vi "TestHB_Emb_1.vi"() -> ()   [LabVIEW 2012]
doc: "SciScan 1.2 160622"
uses:
  SubVIs/Heartbeat state manager Input VI names.ctl
  Custom Controls and Typedefs/HFG Commands.ctl
  Custom Controls/Heartbeat_States.ctl
  Custom Controls and Typedefs/HB Actionable Event.ctl
  Custom Controls and Typedefs/Heartbeat Event Source.ctl
  Custom Controls and Typedefs/Heartbeat information cluster.ctl
  SubVIs/Master Slave messaging Flags.ctl
  Custom Controls and Typedefs/HB_Error Conditions Cluster.ctl
panel:
  out "Commands Sent":i32
  out "No of slave confirmation":i32
  out "Error conditions Cluster":T1
  out "Master-Slave messaging Flags":T2={"Instruction available"=TRUE, "Slave action completed"=TRUE, "Slave Ready?"=FALSE}
  out "Heartbeat information cluster":T3
  in  "stop 3":bool
  in  "stop 2":bool
  out "Commands Issued":i32
  in  "Completion simulator":bool
  in  "Array":string[](array[string])=["Hi", "This", "Is", "A", "Test", "fg", "fgg", "ghg", "gh", "gh", "gh", "h", "hg", "f", "gn", "dghs", "dgh", "dghd", "dh", "d", "dghz", "afd", "gh", "afdg", "adfg", "dafg", "dfgh", "adfg", "dfg", "fdg", "dafg", "a", "hz", "fg", "dafg", "fdg", "adfg", "ag", "hadfg", "dfg", "adfg", "afg", "gjsgh", "dfhg", "dfg", "dfg", "jadfgh", "fhad", "hdgfh", "adfg", "hsdhgf", "adfg", "hdgfh", "fgg", "hdafh", "fdghfd", "hgsdha", "adfga", "ghadfh", "fdh", "fhjda", "fgasd", "hdha", "ahfdjhs", "dha", "hjg", "jgfsj", "adgh", "sdgh", "dsgjs", "adfh", "sdgha", "fdha", "dfhhs", "hgshjs", "gjhs", "gdh", "sgfh", "sgh", "gjhs", "hfdj", "dsfhj", "dfh", "jdhj", "fhjd", "ghfg", "fhjd", "dfjdf", "hjdf", "gjdfgj", "fhjd", "jkkg", "kfdh", "dfhjsd", "fhj", "fhj", "sfgj", "sfgjsf", "fgjgfj", "sfgjsf", "jfghjsgf", "fghjsf", "fsghj"]
  in  "Cancel simulator":bool
  out "Error Out":errorcluster
  in  "Error In":errorcluster
  in  "Command Issue simulator":bool
  in  "stop":bool
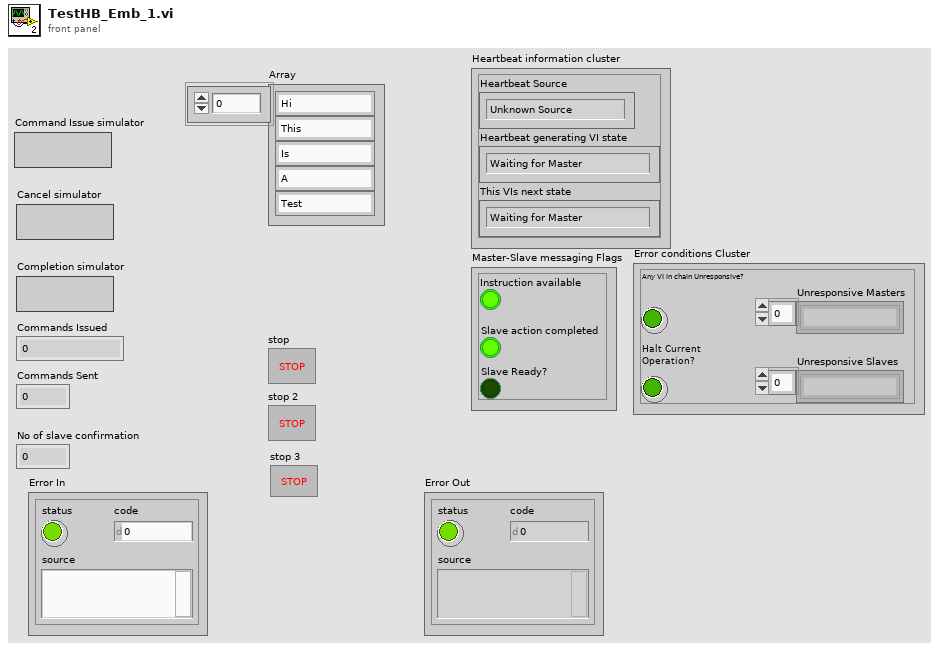
[diagram p1: front panel]
types:
  T1 = typedef "HB_Error Conditions Cluster.ctl" = cluster{"Any VI in chain Unresponsive?":bool, "Halt Current Operation?":bool, "Unresponsive Masters":string[], "Unresponsive Slaves":string[]}
  T2 = typedef "Master Slave messaging Flags.ctl" = cluster{"Instruction available":bool, "Slave action completed":bool, "Slave Ready?":bool}
  T3 = typedef "Heartbeat information cluster.ctl" = cluster{"Heartbeat Source":T4, "Heartbeat generating VI state":T5, "This VIs next state":T5}
  T4 = typedef "Heartbeat Event Source.ctl" = enum16{"Unknown Source", "Timeout", "This VI", "Master", "Slave"}
  T5 = typedef "Heartbeat_States.ctl" = enum16{"Waiting for Master", "Instruction Issued", "Waiting for Slave Completion", "Completed", "Cancelled", "Failed", "Broken Link"}
  T6 = enum8{"Enabled", "Disabled", "Disabled and Grayed Out"}
  T7 = typedef "HB Actionable Event.ctl" = enum16{"Master instruction event", "Slave ready event", "Slave unavailable event", "Cancelled or Failed event", "Slave action complete event", "QUIT", "Broken Link", "Recovered from Broken Link"}
  T8 = typedef "Heartbeat state manager Input VI names.ctl" = cluster{"Current VI name":string, "Master VI Names":string[], "Slave VI Names":string[]}
  T9 = typedef "HFG Commands.ctl" = enum16{"Set", "Get", "Initialize"}
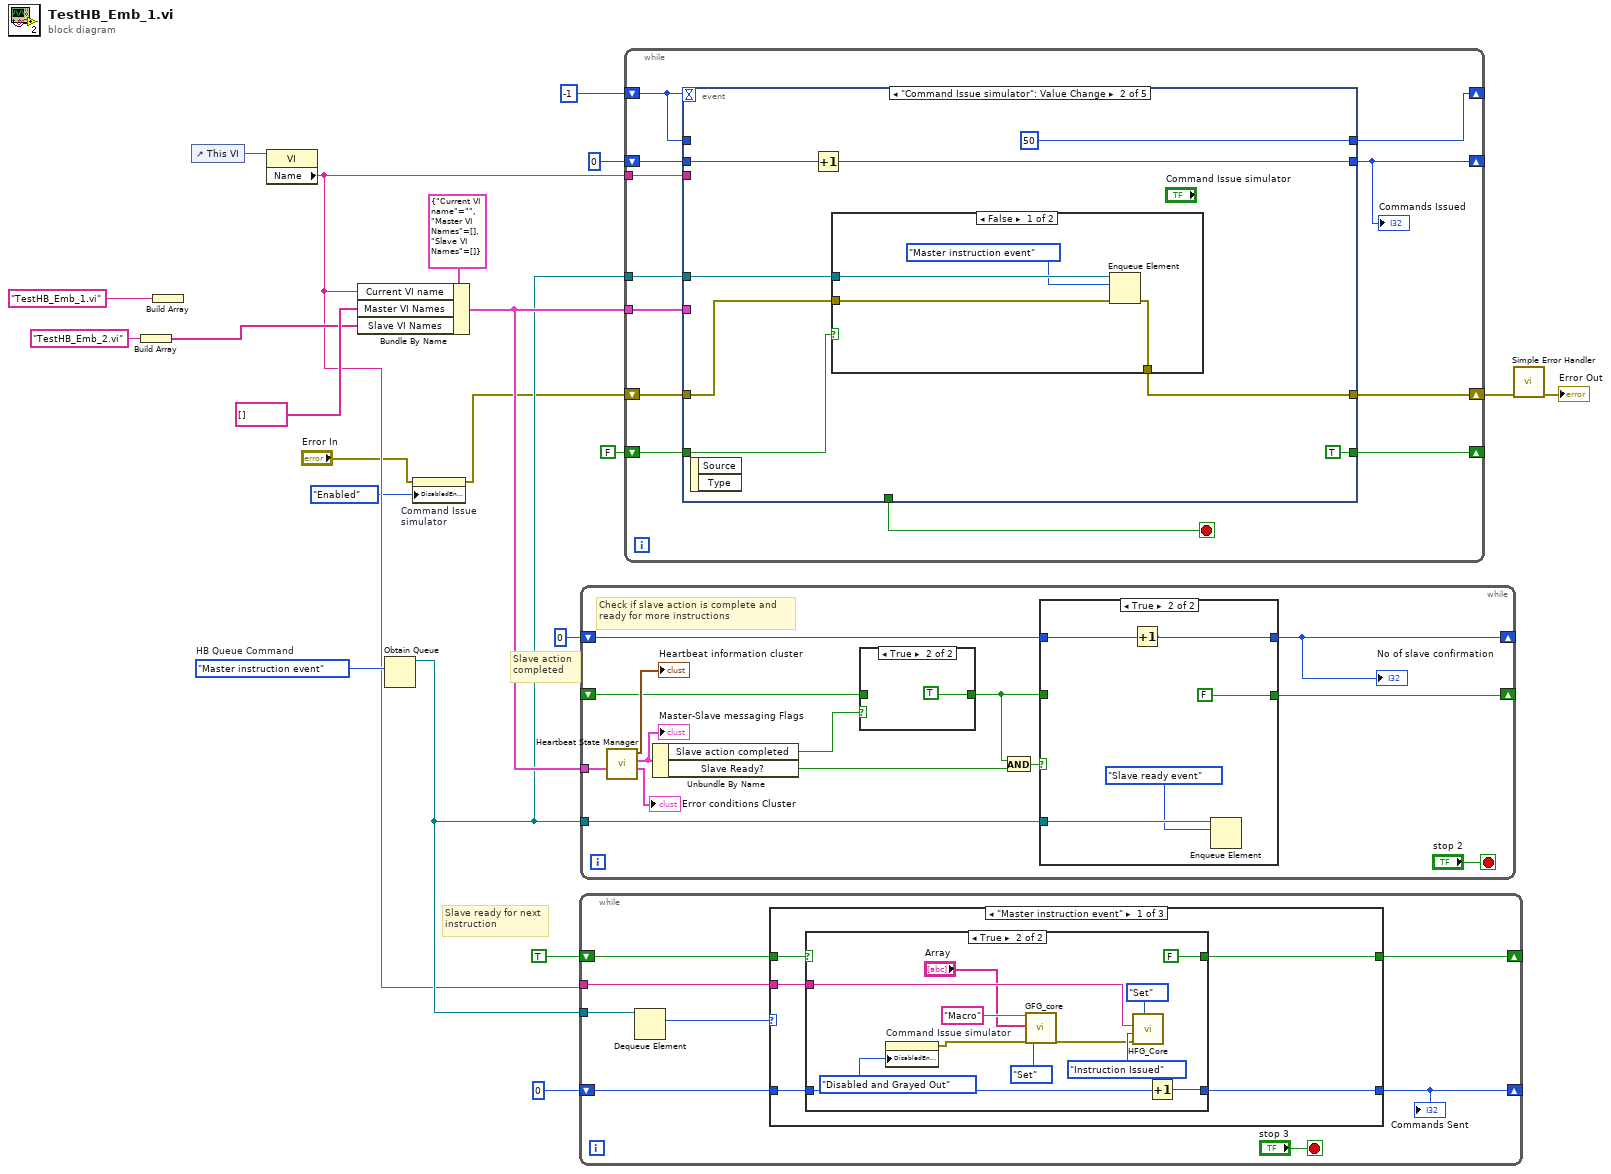
[diagram p0: block diagram]
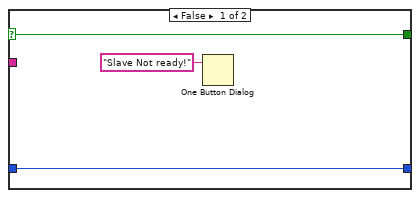
[diagram p2: hidden frame]
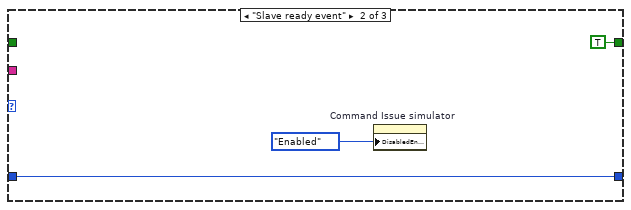
[diagram p3: hidden frame]
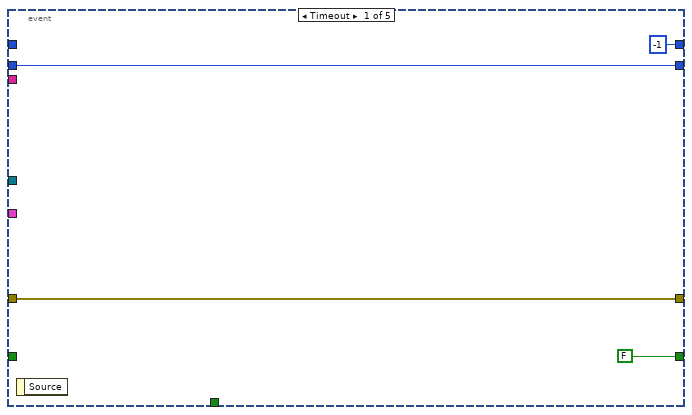
[diagram p7: hidden frame]
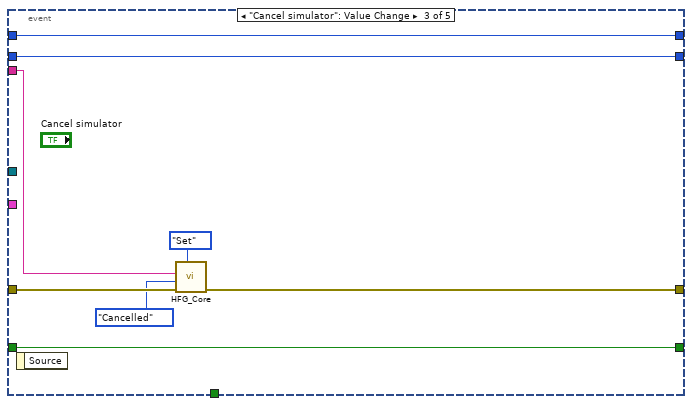
[diagram p9: hidden frame]
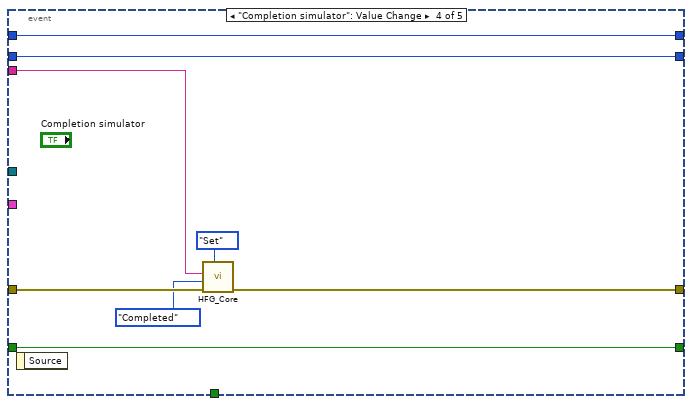
[diagram p10: hidden frame]
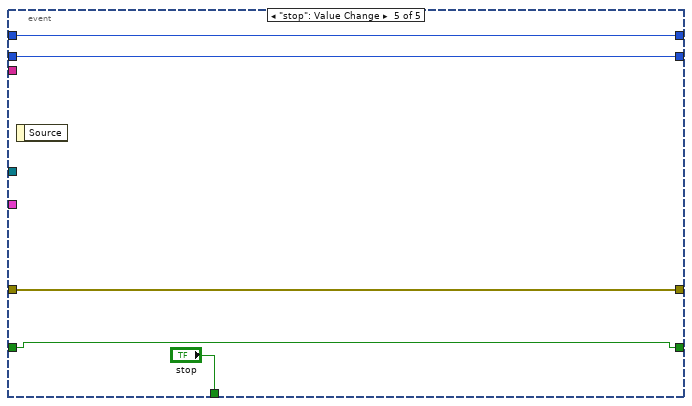
[diagram p11: hidden frame]
diagram:
  w12 = HB_Actionable_Event."Master instruction event"  # HB Queue Command
  # "Slave action \ncompleted"
  # "Slave ready for next\ninstruction"
  n1 = Build Array("TestHB_Emb_2.vi") -> (w17:string[])
  n2 = Build Array("TestHB_Emb_1.vi") -> ()  [unwired: 1 out]
  n3 = control-ref of="This VI"() -> (w16:refnum<vi>)
  n4 = property class="VI"(reference=w16) -> ("Name"=w10:string)  [unwired: 1 in, 2 out]
  n5 = Bundle By Name(cluster=T8 {"Current VI name"="", "Master VI Names"=[], "Slave VI Names"=[]} ("Heartbeat state manager Input VI names 2"), "Current VI name"=w10, "Master VI Names"=string[] [], "Slave VI Names"=w17) -> (w13:T8)
  n6 = Obtain Queue(element data type=w12) -> (queue out=w11:refnum<queue>)  [unwired: 4 in, 2 out]
  n7 = property on="Command Issue simulator" class="Bool"(error in="Error In", "DisabledEnum"=T6."Enabled" ("Disabled")) -> (error out=w7:errorcluster)  [unwired: 1 in, 1 out]
  n8 = while {
    tunnel: w11 -> [w29]
    tunnel: w10 -> [w26]
    shift-right: [w25] -> _
    shift-left: TRUE -> [w24]
    shift-right: [w22] -> _
    shift-left: 0 -> [w23]
    stop <- "stop 3" stop-if-true
    n9 = Dequeue Element(queue=w29) -> (element=w28:T7)  [unwired: 2 in, 3 out]
    n10 = case shown="\"Master instruction event\"" w28 {
      tunnel: w26 -> [w34 _ _]
      tunnel: [w32 TRUE w54] -> w25
      tunnel: w24 -> [w33 _ w54]
      tunnel: w23 -> [w31 w50 w53]
      tunnel: [w30 w50 w53] -> w22
      frame "Master instruction event" {
        n11 = case shown="True" w33 {
          selector: w33 -> [w36 _]
          tunnel: w34 -> [_ w49]
          tunnel: [w36 FALSE] -> w32
          tunnel: w31 -> [w35 w39]
          tunnel: [w35 w38] -> w30
          frame False {
            n12 = One Button Dialog(message="Slave Not ready!") -> ()  [unwired: 1 in, 1 out]
          }
          frame True {
            n13 = property on="Command Issue simulator" class="Bool"("DisabledEnum"=T6."Disabled and Grayed Out" ("Disabled")) -> (error out=w40:errorcluster)  [unwired: 2 in, 1 out]
            n14 = call "GFG_core.vi"("Variable Name in"="Macro", "Variant in"="Array", "error in (no error)"=w40, "Action"=enum16{"Init", "Set", "Get", "Clear"}."Set") -> ("error out"=w46:errorcluster)  [unwired: 9 in, 6 out]
            n15 = call "HFG_Core.vi"("HFG Commands"=HFG_Commands."Set", "Error In"=w46, "Heartbeat state IN"=Heartbeat_States."Instruction Issued", "VI Name (Calling VIs name by default)"=w49) -> ()  [unwired: 4 in, 4 out]
            n16 = Increment(x=w39) -> (x+1=w38:i32)
          }
        }
      }
      frame "Slave ready event" {
        n17 = property on="Command Issue simulator" class="Bool"("DisabledEnum"=T6."Enabled" ("Disabled")) -> ()  [unwired: 2 in, 2 out]
      }
      frame Default {
      }
    }
    "Commands Sent" <- w22
  }
  n18 = while {
    tunnel: w13 -> [w67]
    tunnel: w11 -> [w58]
    shift-right: [w55] -> _
    shift-left: 0 -> [w56]
    shift-right: [w57] -> _
    shift-left: _ -> [w62]
    stop <- "stop 2" stop-if-true
    # "Check if slave action is complete and ready for more instructions"
    n19 = call "Heartbeat State Manager.vi"("Heartbeat state manager Input VI names"=w67) -> ("Error conditions Cluster"=→"Error conditions Cluster":T1, "Master-Slave messaging Flags"=w66:T2, "Heartbeat information cluster"=→"Heartbeat information cluster":T3)  [unwired: 5 in, 3 out]
    "Master-Slave messaging Flags" <- w66
    n20 = Unbundle By Name(w66) -> ("Slave action completed"=w63:bool, "Slave Ready?"=w61:bool)
    n21 = case shown="True" w63 {
      tunnel: [w76 TRUE] -> w60
      tunnel: w62 -> [w76 _]
      frame False {
      }
      frame True {
      }
    }
    n22 = And(x=w60, y=w61) -> (x .and. y?=w59:bool)
    n23 = case shown="True" w59 {
      tunnel: w60 -> [w69 _]
      tunnel: w58 -> [_ w75]
      tunnel: [w69 FALSE] -> w57
      tunnel: w56 -> [w70 w73]
      tunnel: [w70 w72] -> w55
      frame False {
      }
      frame True {
        n24 = Increment(x=w73) -> (x+1=w72:i32)
        n25 = Enqueue Element(queue=w75, element=HB_Actionable_Event."Slave ready event") -> ()  [unwired: 2 in, 3 out]
      }
    }
    "No of slave confirmation" <- w55
  }
  n26 = while {
    tunnel: w13 -> [w87]
    shift-right: [w86] -> w15
    shift-left: w7 -> [w88]
    tunnel: w10 -> [w85]
    tunnel: w11 -> [w84]
    shift-right: [w82] -> _
    shift-left: 0 -> [w83]
    shift-right: [w81] -> _
    shift-left: -1 -> [w80]
    shift-right: [w79] -> _
    shift-left: FALSE -> [w78]
    stop <- w89 stop-if-true
    n27 = event shown="[1] \"Command Issue simulator\": Value Change" {
      selector: _ -> [_ _ _ _ _]
      dyn-events: _ -> [_ _ _ _ _]
      timeout: w80 -> [_ _ _ _ _]
      tunnel: [_ _ _ _ "stop"] -> w89
      tunnel: w88 -> [w93 w99 w114 w122 w126]
      tunnel: w87 -> [_ _ _ _ _]
      tunnel: [w93 w100 w110 w118 w126] -> w86
      tunnel: w85 -> [_ _ w112 w120 _]
      tunnel: w84 -> [_ w101 _ _ _]
      tunnel: w83 -> [w92 w98 w109 w117 w125]
      tunnel: [w92 w97 w109 w117 w125] -> w82
      tunnel: [-1 50 w108 w116 w124] -> w81
      tunnel: w80 -> [_ _ w108 w116 w124]
      tunnel: [FALSE TRUE w107 w115 w123] -> w79
      tunnel: w78 -> [_ w94 w107 w115 w123]
      event Timeout {
        n28 = event-data() -> ()  [unwired: 1 in, 1 out]
      }
      event "Command Issue simulator": Value Change {
        n29 = event-data() -> ()  [unwired: 1 in, 2 out]
        n30 = Increment(x=w98) -> (x+1=w97:i32)
        n31 = case shown="False" w94 {
          tunnel: w101 -> [w105 _]
          tunnel: [w103 w106] -> w100
          tunnel: w99 -> [w102 w106]
          frame False {
            n32 = Enqueue Element(queue=w105, element=HB_Actionable_Event."Master instruction event", error in (no error)=w102) -> (error out=w103:errorcluster)  [unwired: 1 in, 2 out]
          }
          frame True {
            # "Multiple presses detected - ignore!"
          }
        }
      }
      event "Cancel simulator": Value Change {
        n33 = event-data() -> ()  [unwired: 1 in, 1 out]
        n34 = call "HFG_Core.vi"("HFG Commands"=HFG_Commands."Set", "Error In"=w114, "Heartbeat state IN"=Heartbeat_States."Cancelled", "VI Name (Calling VIs name by default)"=w112) -> ("Error Out"=w110:errorcluster)  [unwired: 4 in, 3 out]
      }
      event "Completion simulator": Value Change {
        n35 = event-data() -> ()  [unwired: 1 in, 1 out]
        n36 = call "HFG_Core.vi"("HFG Commands"=HFG_Commands."Set", "Error In"=w122, "Heartbeat state IN"=Heartbeat_States."Completed", "VI Name (Calling VIs name by default)"=w120) -> ("Error Out"=w118:errorcluster)  [unwired: 4 in, 3 out]
      }
      event "stop": Value Change {
        n37 = event-data() -> ()  [unwired: 1 in, 1 out]
      }
    }
    "Commands Issued" <- w82
  }
  n38 = call <vilib>:"Simple Error Handler.vi"("error in (no error)"=w15) -> ("error out"=→"Error Out":errorcluster)  [unwired: 4 in, 4 out]
